vi "writeTest.vi"   [LabVIEW 2015]
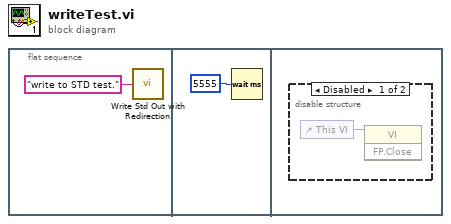
[diagram p0: block diagram]
diagram:
  n1 = flat-sequence {
    frame #0 {
      n2 = call "Write Std Out with Redirection.vi"("text"="write to STD test.") -> ()
    }
    frame #1 {
      n3 = Wait (ms)(milliseconds to wait=u32 5555) -> ()  [unwired: 1 out]
    }
    frame #2 {
      n4 = disable-structure shown="Disabled" {
        frame Disabled {
          n5 = control-ref of="This VI"() -> (w3:refnum<vi>)
          n6 = invoke class="VI" method="FP.Close"(reference=w3) -> ()  [unwired: 2 in, 3 out]
        }
        frame Enabled {
        }
      }
    }
  }
